vi "_PC_InterfaceToolbar signalReceptionCommand.vi"() -> ()   [LabVIEW 2018]
panel:
  out "MSAnalExe?":bool
  out "ExeTimes Out":i32
  in  "Loops in":i32
  in  "dataManagRefnum":T1
  out "error out":errorcluster
  in  "error in (no error)":errorcluster
  in  "actionCmd":T2
  in  "function":T3(ring)
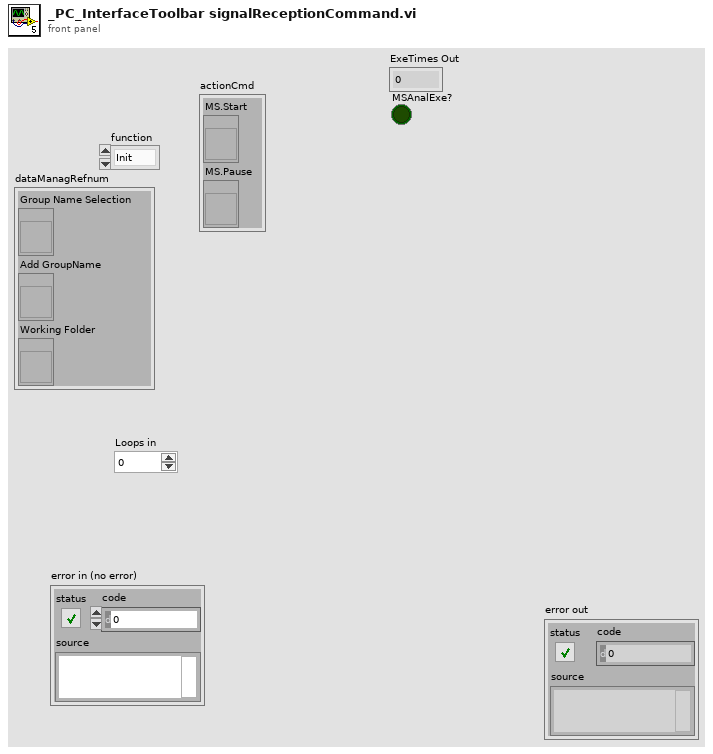
[diagram p1: front panel]
types:
  T1 = cluster{"Group Name Selection":refnum<vi>, "Add GroupName":refnum<vi>, "Working Folder":refnum<vi>}
  T2 = cluster{"MS.Start":refnum<vi>, "MS.Pause":refnum<vi>}
  T3 = enum16{"Init", "Start", "StartInf", "Pause", "Queue"}
  T4 = cluster{"MassAnalExe?":refnum<k21>, "MassAnalPause":refnum<k21>, "MassAnalExe":refnum<k21>, "ExeTimes":refnum<k21>}
  T5 = enum8{"Enabled", "Disabled", "Disabled and Grayed Out"}
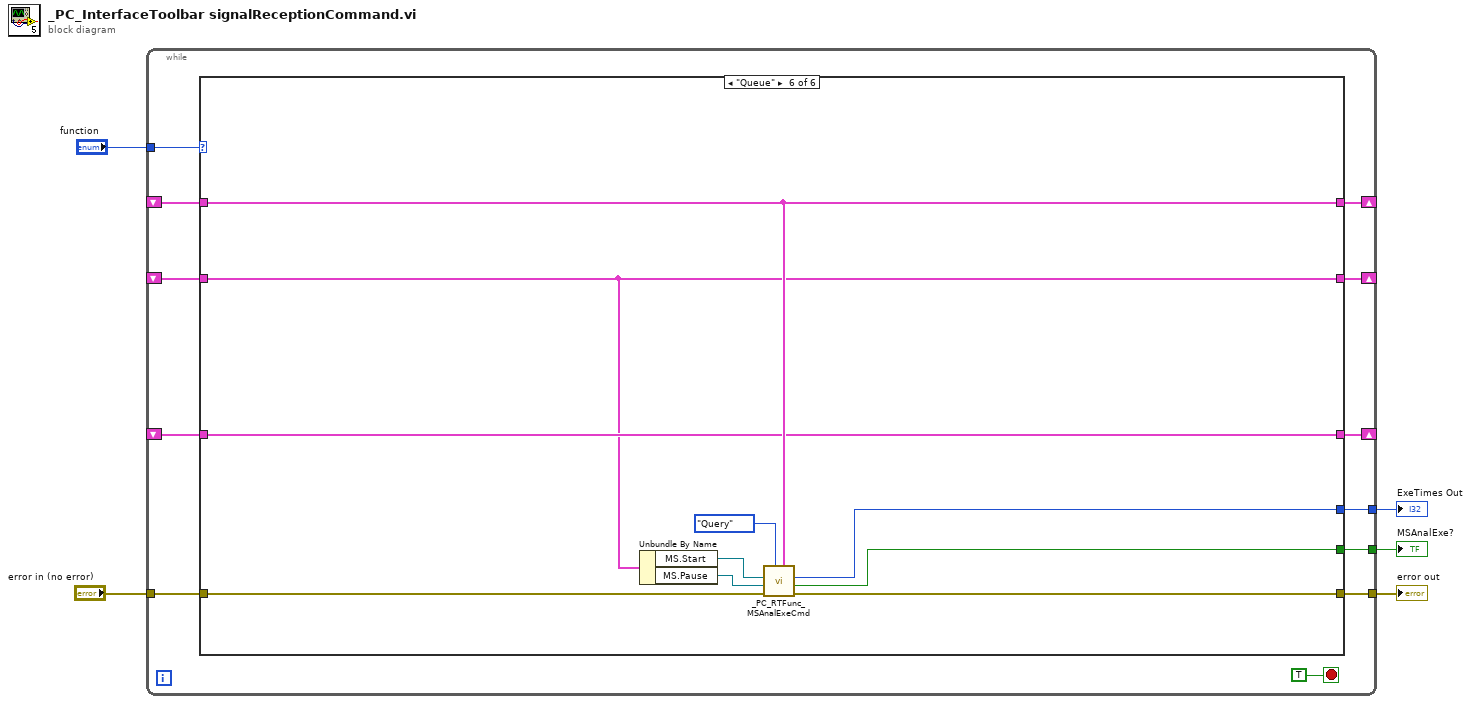
[diagram p0: block diagram]
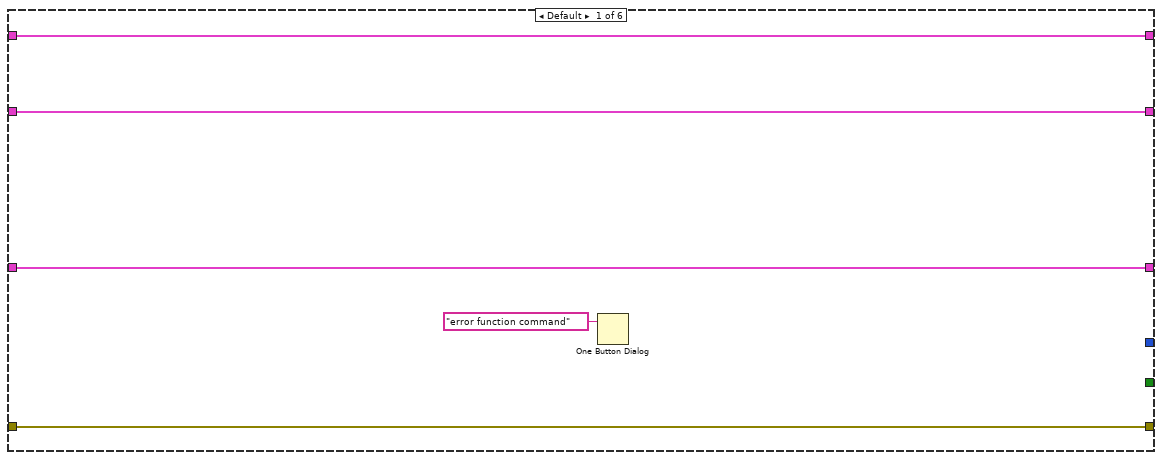
[diagram p2: hidden frame]
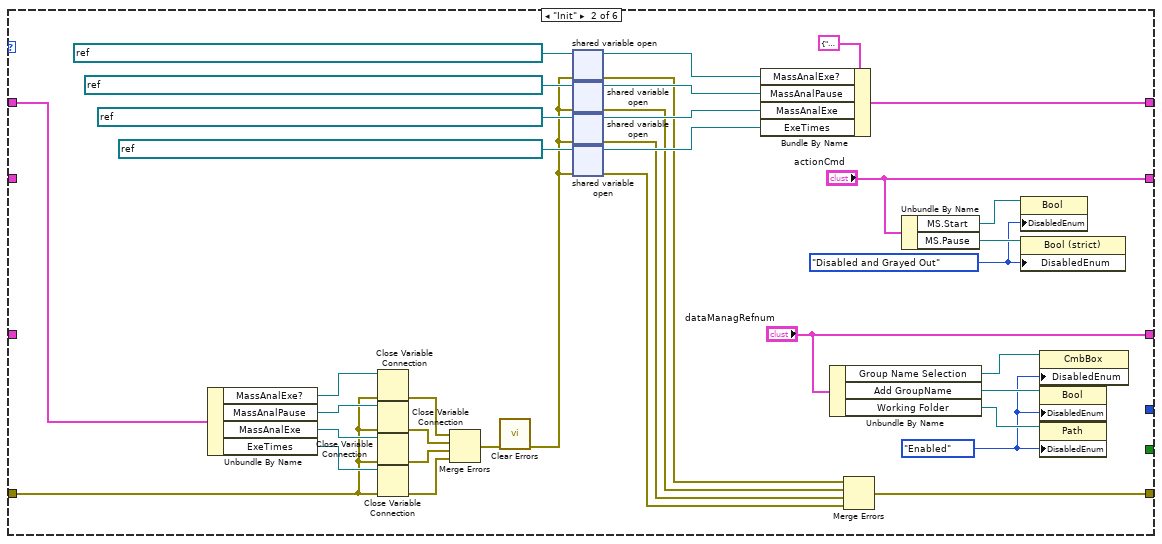
[diagram p3: hidden frame]
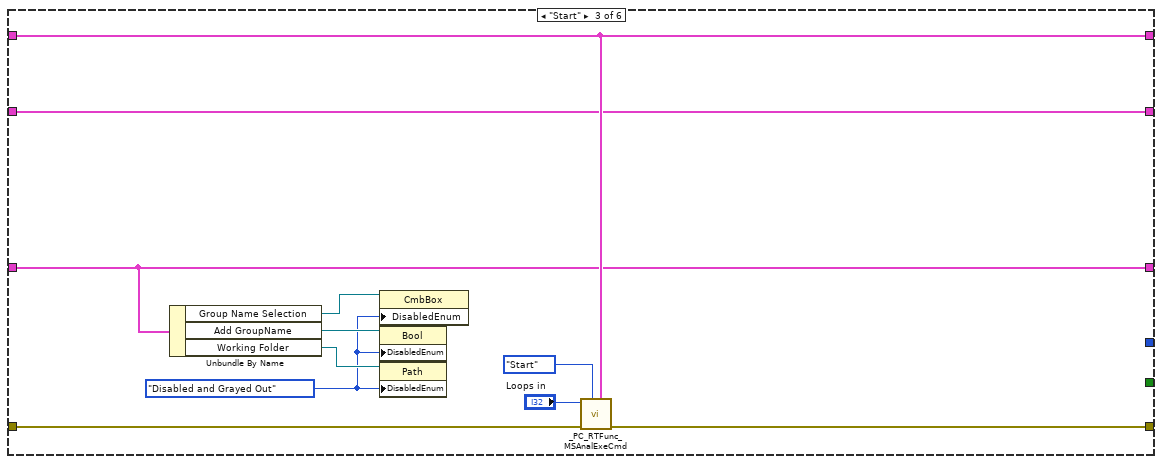
[diagram p4: hidden frame]
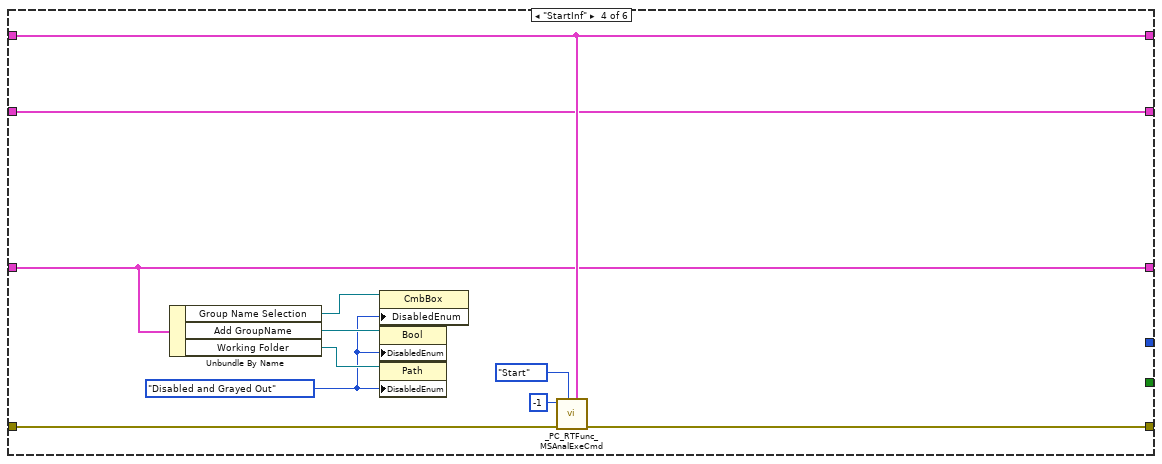
[diagram p5: hidden frame]
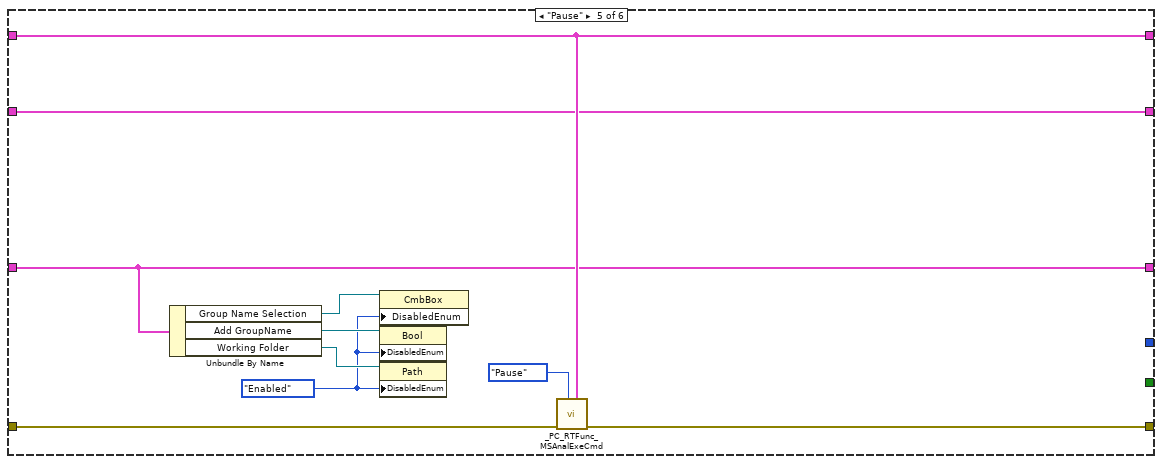
[diagram p6: hidden frame]
diagram:
  n1 = while {
    tunnel: "function" -> [w17]
    shift-right: [w16] -> _
    shift-left: _ -> [w15]
    tunnel: "error in (no error)" -> [w14]
    tunnel: [w13] -> w3
    shift-right: [w12] -> _
    shift-left: _ -> [w11]
    shift-right: [w10] -> _
    shift-left: _ -> [w8]
    tunnel: [w7] -> w2
    tunnel: [w6] -> w1
    stop <- TRUE stop-if-true
    n2 = case shown="\"Queue\"" w17 {
      tunnel: [w21 w36 w67 w78 w88 w98] -> w16
      tunnel: w15 -> [w21 w35 w67 w78 w88 w98]
      tunnel: w14 -> [w22 w31 w69 w80 w90 w100]
      tunnel: [w22 w30 w68 w79 w89 w99] -> w13
      tunnel: [w20 "actionCmd" w66 w77 w87 w95] -> w12
      tunnel: w11 -> [w20 _ w66 w77 w87 w95]
      tunnel: [w19 "dataManagRefnum" w61 w72 w82 w97] -> w10
      tunnel: w8 -> [w19 _ w61 w72 w82 w97]
      tunnel: [_ _ _ _ _ w92] -> w7
      tunnel: [_ _ _ _ _ w91] -> w6
      frame Default {
        n3 = One Button Dialog(message="error function command") -> ()  [unwired: 1 in, 1 out]
      }
      frame "Init" {
        w23 = T5."Enabled" ("Disabled")
        w28 = T5."Disabled and Grayed Out" ("Disabled")
        n4 = Unbundle By Name(w35) -> ("MassAnalExe?"=w39:refnum<k21>, "MassAnalPause"=w45:refnum<k21>, "MassAnalExe"=w44:refnum<k21>, "ExeTimes"=w43:refnum<k21>)
        n5 = Close Variable Connection(8:w31, 11:w39) -> (0:w42:errorcluster)
        n6 = Close Variable Connection(8:w31, 11:w45) -> (0:w41:errorcluster)
        n7 = Close Variable Connection(8:w31, 11:w44) -> (0:w40:errorcluster)
        n8 = Close Variable Connection(8:w31, 11:w43) -> (0:w37:errorcluster)
        n9 = Merge Errors(w42, w41, w40, w37) -> (w38:errorcluster)
        n10 = call <vilib>:"Clear Errors.vi"("error in (no error)"=w38) -> ("error out"=w34:errorcluster)  [unwired: 5 in, 1 out]
        n11 = shared-variable-open(refnum<k21> "ni.var.psp://NI-sbRIO/_RT_CtrlLoop_MassAnalysing_Variable/MassAnalExe%3F" ("shared variable refnum in"), w34) -> (w55:refnum<k21>, w49:errorcluster)
        n12 = shared-variable-open(refnum<k21> "ni.var.psp://NI-sbRIO/_RT_CtrlLoop_MassAnalysing_Variable/MassAnalPause" ("shared variable refnum in"), w34) -> (w56:refnum<k21>, w48:errorcluster)
        n13 = shared-variable-open(refnum<k21> "ni.var.psp://NI-sbRIO/_RT_CtrlLoop_MassAnalysing_Variable/MassAnalExe" ("shared variable refnum in"), w34) -> (w57:refnum<k21>, w47:errorcluster)
        n14 = shared-variable-open(refnum<k21> "ni.var.psp://NI-sbRIO/_RT_CtrlLoop_MassAnalysing_Variable/ExeTimes" ("shared variable refnum in"), w34) -> (w58:refnum<k21>, w46:errorcluster)
        n15 = Bundle By Name(cluster=T4 {"MassAnalExe?"="", "MassAnalPause"="", "MassAnalExe"="", "ExeTimes"=""} ("connectStateSV"), "MassAnalExe?"=w55, "MassAnalPause"=w56, "MassAnalExe"=w57, "ExeTimes"=w58) -> (w36:T4)
        n16 = Unbundle By Name("dataManagRefnum") -> ("Group Name Selection"=w26:refnum<vi>, "Add GroupName"=w25:refnum<vi>, "Working Folder"=w24:refnum<vi>)
        n17 = Merge Errors(w49, w48, w47, w46) -> (w30:errorcluster)
        n18 = Unbundle By Name("actionCmd") -> ("MS.Start"=w33:refnum<vi>, "MS.Pause"=w32:refnum<vi>)
        n19 = property class="Bool"(reference=w33, "DisabledEnum"=w28) -> ()  [unwired: 1 in, 2 out]
        n20 = property class="Bool (strict)"(reference=w32, "DisabledEnum"=w28) -> ()  [unwired: 1 in, 2 out]
        n21 = property class="CmbBox"(reference=w26, "DisabledEnum"=w23) -> ()  [unwired: 1 in, 2 out]
        n22 = property class="Bool"(reference=w25, "DisabledEnum"=w23) -> ()  [unwired: 1 in, 2 out]
        n23 = property class="Path"(reference=w24, "DisabledEnum"=w23) -> ()  [unwired: 1 in, 2 out]
      }
      frame "Start" {
        w62 = T5."Disabled and Grayed Out" ("Disabled")
        n24 = Unbundle By Name(w61) -> ("Group Name Selection"=w65:refnum<vi>, "Add GroupName"=w64:refnum<vi>, "Working Folder"=w63:refnum<vi>)
        n25 = property class="CmbBox"(reference=w65, "DisabledEnum"=w62) -> ()  [unwired: 1 in, 2 out]
        n26 = property class="Bool"(reference=w64, "DisabledEnum"=w62) -> ()  [unwired: 1 in, 2 out]
        n27 = property class="Path"(reference=w63, "DisabledEnum"=w62) -> ()  [unwired: 1 in, 2 out]
        n28 = call "_PC_RTFunc_MSAnalExeCmd.vi"("sv refnum"=w67, "Function"=enum16{"Query", "Start", "Pause"}."Start", "error in (no error)"=w69, "Loops in"="Loops in") -> ("error out"=w68:errorcluster)  [unwired: 5 in, 2 out]
      }
      frame "StartInf" {
        w73 = T5."Disabled and Grayed Out" ("Disabled")
        n29 = Unbundle By Name(w72) -> ("Group Name Selection"=w76:refnum<vi>, "Add GroupName"=w75:refnum<vi>, "Working Folder"=w74:refnum<vi>)
        n30 = property class="CmbBox"(reference=w76, "DisabledEnum"=w73) -> ()  [unwired: 1 in, 2 out]
        n31 = property class="Bool"(reference=w75, "DisabledEnum"=w73) -> ()  [unwired: 1 in, 2 out]
        n32 = property class="Path"(reference=w74, "DisabledEnum"=w73) -> ()  [unwired: 1 in, 2 out]
        n33 = call "_PC_RTFunc_MSAnalExeCmd.vi"("sv refnum"=w78, "Function"=enum16{"Query", "Start", "Pause"}."Start", "error in (no error)"=w80, "Loops in"=-1) -> ("error out"=w79:errorcluster)  [unwired: 5 in, 2 out]
      }
      frame "Pause" {
        w83 = T5."Enabled" ("Disabled")
        n34 = Unbundle By Name(w82) -> ("Group Name Selection"=w86:refnum<vi>, "Add GroupName"=w85:refnum<vi>, "Working Folder"=w84:refnum<vi>)
        n35 = property class="CmbBox"(reference=w86, "DisabledEnum"=w83) -> ()  [unwired: 1 in, 2 out]
        n36 = property class="Bool"(reference=w85, "DisabledEnum"=w83) -> ()  [unwired: 1 in, 2 out]
        n37 = property class="Path"(reference=w84, "DisabledEnum"=w83) -> ()  [unwired: 1 in, 2 out]
        n38 = call "_PC_RTFunc_MSAnalExeCmd.vi"("sv refnum"=w88, "Function"=enum16{"Query", "Start", "Pause"}."Pause", "error in (no error)"=w90) -> ("error out"=w89:errorcluster)  [unwired: 6 in, 2 out]
      }
      frame "Queue" {
        n39 = Unbundle By Name(w95) -> ("MS.Start"=w93:refnum<vi>, "MS.Pause"=w94:refnum<vi>)
        n40 = call "_PC_RTFunc_MSAnalExeCmd.vi"("sv refnum"=w98, "Function"=enum16{"Query", "Start", "Pause"}."Query", "error in (no error)"=w100, "MS.Pause"=w94, "MS.Start"=w93) -> ("error out"=w99:errorcluster, "MSAnalExe?"=w91:bool, "ExeTimes Out"=w92:i32)  [unwired: 4 in]
      }
    }
  }
  "error out" <- w3
  "ExeTimes Out" <- w2
  "MSAnalExe?" <- w1
